vi "用户管理.vi"(6 "用户名的顺序":u16, 8 "用户类别":u8, 9 "管理人员1+密码":string[][](array[string]), 10 "操作人员0+密码":string[][](array[string]), 11 "密码文件路径":path=path "E:/LabVIEW Data/盾构/default") -> (0 "用户类别-out":u8, 1 "管理人员1+密码-out":string[][](array[string]), 2 "操作人员0+密码-out":string[][](array[string]), 3 "用户信息":string, 5 "用户名的顺序-out":u16)   [LabVIEW 2018]
panel:
  out "数值-当前用户名":u16
  out "数值-当前用户类别":u8
  in  "切换用户":bool
  in  "返回":bool
  in  "修改密码":bool
  in  "删除":bool
  in  "增加":bool
  in  "请输入密码":string
  in  "用户名":u16(ring) items=["1", "2"]
  in  "用户类别":u8(ring) items=["操作人员", "管理人员"]
  out "当前用户类别":string
  out "当前用户名":string
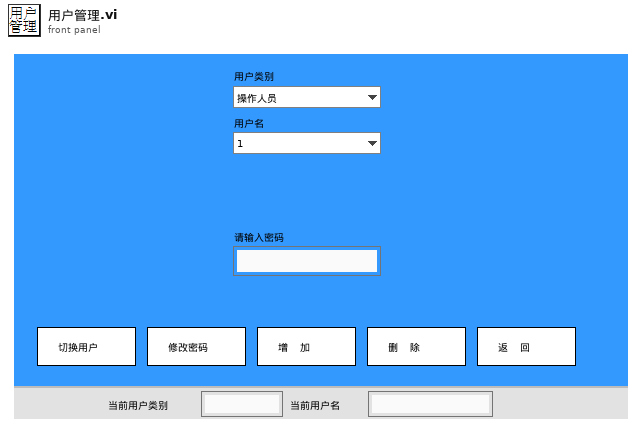
[diagram p1: front panel]
types:
  T1 = cluster{"数值-当前用户类别":u8, "当前用户类别":string, "数值-当前用户名":u16, "当前用户名":string}
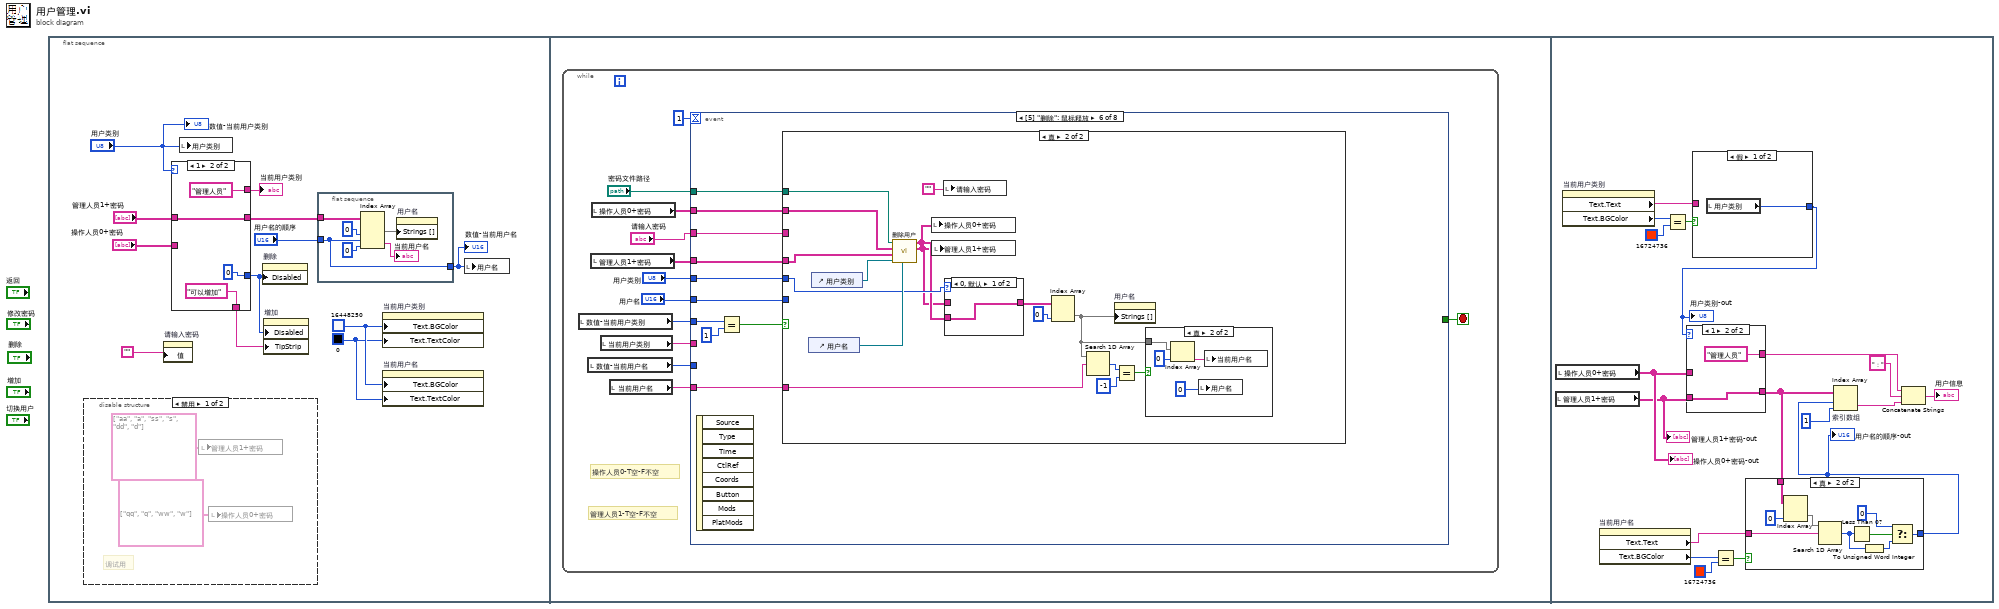
[diagram p0: block diagram]
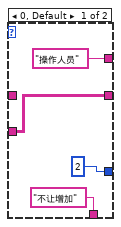
[diagram p3: hidden frame]
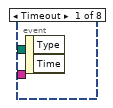
[diagram p4: hidden frame]
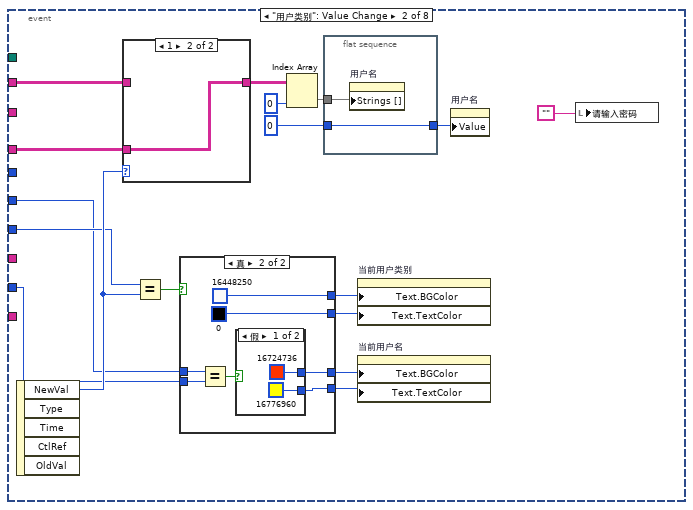
[diagram p5: hidden frame]
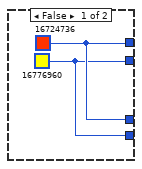
[diagram p6: hidden frame]
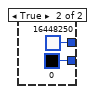
[diagram p7: hidden frame]
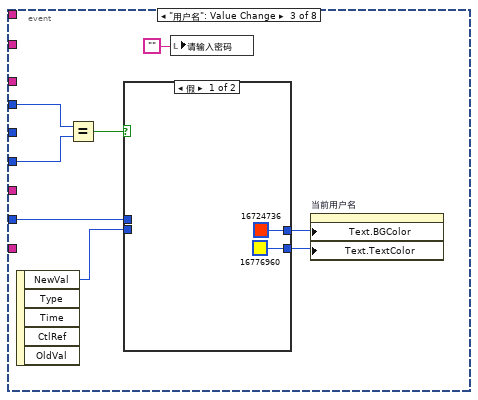
[diagram p9: hidden frame]
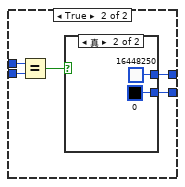
[diagram p10: hidden frame]
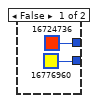
[diagram p11: hidden frame]
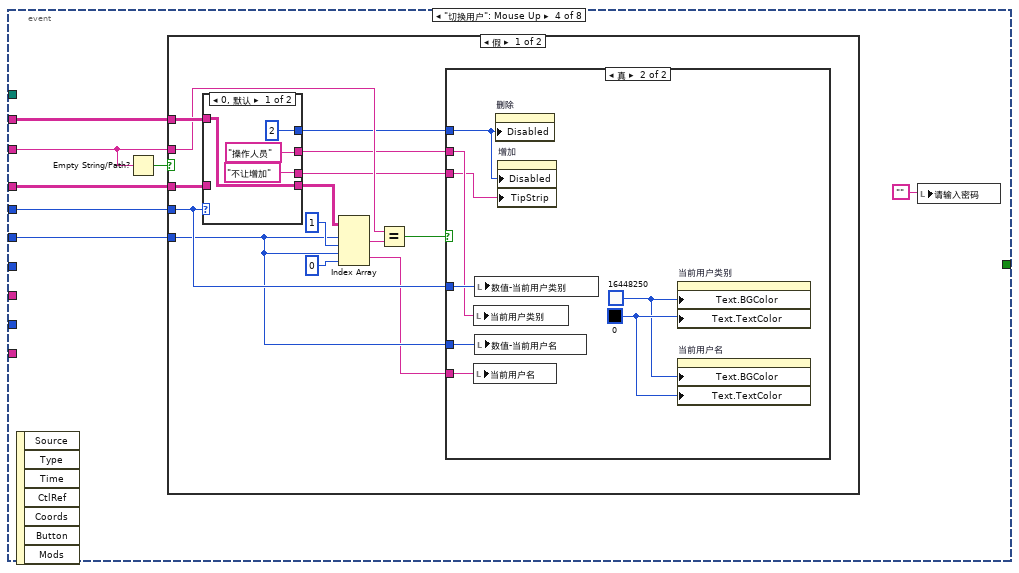
[diagram p12: hidden frame]
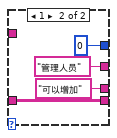
[diagram p14: hidden frame]
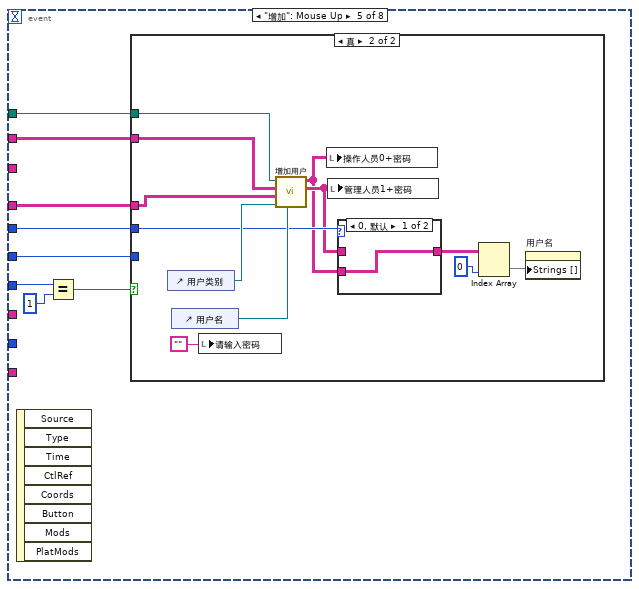
[diagram p16: hidden frame]
diagram:
  n1 = flat-sequence {
    frame #0 {
      w3 = u32 16448250 ("前")
      w2 = u32 0 ("颜色盒")
      n2 = disable-structure shown="禁用" {
        frame Disabled {
          # "调试用"
          n3 = local write "管理人员1+密码"(string[][] [["aa", "a"], ["ss", "s"], ["dd", "d"]] ("管理人员1+密码")) -> ()
          n4 = local write "操作人员0+密码"(string[][] [["qq", "q"], ["ww", "w"]] ("管理人员1+密码")) -> ()
        }
        frame Enabled {
        }
      }
      n5 = property on="请输入密码" class="Str"("值"="") -> ()  [unwired: 2 in, 2 out]
      n6 = case shown="1" "用户类别" {
        tunnel: ["操作人员" "管理人员"] -> w11
        tunnel: "管理人员1+密码" -> [_ w27]
        tunnel: [w23 w27] -> w10
        tunnel: "操作人员0+密码" -> [w23 _]
        tunnel: [u8 2 ("禁用") u8 0 ("禁用")] -> w6
        tunnel: ["不让增加" "可以增加"] -> w1
        frame 0, Default {
        }
        frame 1 {
        }
      }
      "当前用户类别" <- w11
      n7 = local write "用户类别"("用户类别") -> ()
      n8 = property on="删除" class="Bool (严格)"("Disabled"=w6) -> ()  [unwired: 2 in, 2 out]
      n9 = property on="增加" class="Bool (严格)"("Disabled"=w6, "TipStrip"=w1) -> ()  [unwired: 2 in, 2 out]
      n10 = flat-sequence {
        tunnel: w10 -> [w19]
        tunnel: "用户名的顺序" -> [w15]
        tunnel: [w15] -> w8
        frame #0 {
          n11 = Index Array(array=w19, index (col) #1=0 ("禁用的索引 (col)"), index (row) #2=w15, index (col) #2=0 ("禁用的索引 (col)")) -> (element #1=w17:string[], element #2=→"当前用户名":string)  [unwired: 1 in]
          n12 = property on="用户名" class="Ring (严格)"("Strings []"=w17) -> ()  [unwired: 2 in, 2 out]
        }
      }
      n13 = property on="当前用户类别" class="字符串"("Text.BGColor"=w3, "Text.TextColor"=w2) -> ()  [unwired: 2 in, 2 out]
      n14 = property on="当前用户名" class="字符串"("Text.BGColor"=w3, "Text.TextColor"=w2) -> ()  [unwired: 2 in, 2 out]
      n15 = local write "用户名"(w8) -> ()
      "数值-当前用户类别" <- "用户类别"
      "数值-当前用户名" <- w8
    }
    frame #1 {
      n16 = while {
        stop <- w40 stop-if-true
        # "管理人员1-T空-F不空"
        # "操作人员0-T空-F不空"
        n17 = local read "数值-当前用户类别"() -> (w33:u8)
        n18 = local read "数值-当前用户名"() -> (w31:u16)
        n19 = local read "管理人员1+密码"() -> (w36:string[][])
        n20 = local read "操作人员0+密码"() -> (w37:string[][])
        n21 = local read "当前用户类别"() -> (w32:string)
        n22 = local read "当前用户名"() -> (w30:string)
        n23 = event shown="[5] \"删除\": 鼠标释放" {
          selector: _ -> [_ _ _ _ _ _ _ _]
          dyn-events: _ -> [_ _ _ _ _ _ _ _]
          timeout: 1 -> [_ _ _ _ _ _ _ _]
          tunnel: [_ _ _ _ _ _ _ TRUE] -> w40
          tunnel: w37 -> [_ w57 _ w98 w138 w162 w194 _]
          tunnel: w36 -> [_ w54 _ w97 w137 w161 w193 _]
          tunnel: "用户类别" -> [_ _ w78 w100 w136 w160 _ _]
          tunnel: "用户名" -> [_ w43 _ w99 w135 w159 _ _]
          tunnel: "密码文件路径" -> [_ _ _ _ w131 w154 w195 _]
          tunnel: "请输入密码" -> [_ _ _ w96 _ w158 _ _]
          tunnel: w33 -> [_ w49 w77 _ w134 w157 w189 _]
          tunnel: w32 -> [_ _ _ _ _ _ w188 _]
          tunnel: w31 -> [_ w42 w79 _ _ _ w187 _]
          tunnel: w30 -> [_ _ _ _ _ w153 w186 _]
          event Timeout {
            n24 = event-data() -> ()  [unwired: 1 in, 2 out]
          }
          event "用户类别": Value Change {
            n25 = event-data() -> ("NewVal"=w50:u8)  [unwired: 1 in, 4 out]
            n26 = case shown="1" w50 {
              tunnel: w57 -> [w73 _]
              tunnel: [w73 w74] -> w55
              tunnel: w54 -> [_ w74]
              frame 0, Default {
              }
              frame 1 {
              }
            }
            n27 = Equal?(x=w49, y=w50) -> (x = y?=w48:bool)
            n28 = case shown="真" w48 {
              tunnel: [w59 u32 16448250 ("前")] -> w47
              tunnel: [w58 u32 0 ("颜色盒")] -> w46
              tunnel: [w59 w61] -> w45
              tunnel: [w58 w60] -> w44
              tunnel: w43 -> [_ w63]
              tunnel: w42 -> [_ w62]
              frame False {
                w59 = u32 16724736 ("前")
                w58 = u32 16776960 ("颜色盒")
              }
              frame True {
                n29 = Equal?(x=w63, y=w62) -> (x = y?=w64:bool)
                n30 = case shown="假" w64 {
                  tunnel: [u32 16724736 ("前") u32 16448250 ("前")] -> w61
                  tunnel: [u32 16776960 ("颜色盒") u32 0 ("颜色盒")] -> w60
                  frame False {
                  }
                  frame True {
                  }
                }
              }
            }
            n31 = Index Array(array=w55, index (col)=0 ("禁用的索引 (col)")) -> (element=w56:string[])  [unwired: 1 in]
            n32 = flat-sequence {
              tunnel: w56 -> [w72]
              tunnel: [w71] -> w51
              tunnel: u16 0 ("禁用的索引 (col)") -> [w71]
              frame #0 {
                n33 = property on="用户名" class="Ring (严格)"("Strings []"=w72) -> ()  [unwired: 2 in, 2 out]
              }
            }
            n34 = property on="当前用户类别" class="字符串"("Text.BGColor"=w47, "Text.TextColor"=w46) -> ()  [unwired: 2 in, 2 out]
            n35 = property on="当前用户名" class="字符串"("Text.BGColor"=w45, "Text.TextColor"=w44) -> ()  [unwired: 2 in, 2 out]
            n36 = property on="用户名" class="Ring (严格)"("Value"=w51) -> ()  [unwired: 2 in, 2 out]
            n37 = local write "请输入密码"("") -> ()
          }
          event "用户名": Value Change {
            n38 = event-data() -> ("NewVal"=w82:u16)  [unwired: 1 in, 4 out]
            n39 = Equal?(x=w78, y=w77) -> (x = y?=w76:bool)
            n40 = case shown="假" w76 {
              tunnel: w82 -> [_ w89]
              tunnel: [u32 16724736 ("前") w87] -> w81
              tunnel: [u32 16776960 ("颜色盒") w86] -> w80
              tunnel: w79 -> [_ w85]
              frame False {
              }
              frame True {
                n41 = Equal?(x=w85, y=w89) -> (x = y?=w88:bool)
                n42 = case shown="真" w88 {
                  tunnel: [u32 16724736 ("前") u32 16448250 ("前")] -> w87
                  tunnel: [u32 16776960 ("颜色盒") u32 0 ("颜色盒")] -> w86
                  frame False {
                  }
                  frame True {
                  }
                }
              }
            }
            n43 = local write "请输入密码"("") -> ()
            n44 = property on="当前用户名" class="字符串"("Text.BGColor"=w81, "Text.TextColor"=w80) -> ()  [unwired: 2 in, 2 out]
          }
          event "切换用户": Mouse Up {
            n45 = event-data() -> ()  [unwired: 1 in, 7 out]
            n46 = Empty String/Path?(string/path=w96) -> (empty?=w94:bool)
            n47 = case shown="假" w94 {
              tunnel: w100 -> [w107 _]
              tunnel: w99 -> [w105 _]
              tunnel: w98 -> [w114 _]
              tunnel: w97 -> [w113 _]
              tunnel: w96 -> [w109 _]
              frame False {
                n48 = case shown="0, 默认" w107 {
                  tunnel: w114 -> [w126 _]
                  tunnel: w113 -> [_ w130]
                  tunnel: [w126 w130] -> w110
                  tunnel: ["操作人员" "管理人员"] -> w103
                  tunnel: [u8 2 ("禁用") u8 0 ("禁用")] -> w102
                  tunnel: ["不让增加" "可以增加"] -> w101
                  frame 0, Default {
                  }
                  frame 1 {
                  }
                }
                n49 = Index Array(array=w110, index (row) #1=w105, index (col) #1=1 ("禁用的索引 (col)"), index (row) #2=w105, index (col) #2=0 ("禁用的索引 (col)")) -> (element #1=w111:string, element #2=w104:string)
                n50 = Equal?(x=w109, y=w111) -> (x = y?=w108:bool)
                n51 = case shown="真" w108 {
                  tunnel: w107 -> [_ w122]
                  tunnel: w105 -> [_ w121]
                  tunnel: w104 -> [_ w120]
                  tunnel: w103 -> [_ w119]
                  tunnel: w102 -> [_ w116]
                  tunnel: w101 -> [_ w115]
                  frame False {
                  }
                  frame True {
                    w117 = u32 16448250 ("前")
                    w118 = u32 0 ("颜色盒")
                    n52 = local write "当前用户类别"(w119) -> ()
                    n53 = local write "当前用户名"(w120) -> ()
                    n54 = local write "数值-当前用户类别"(w122) -> ()
                    n55 = local write "数值-当前用户名"(w121) -> ()
                    n56 = property on="删除" class="Bool (严格)"("Disabled"=w116) -> ()  [unwired: 2 in, 2 out]
                    n57 = property on="增加" class="Bool (严格)"("Disabled"=w116, "TipStrip"=w115) -> ()  [unwired: 2 in, 2 out]
                    n58 = property on="当前用户类别" class="字符串"("Text.BGColor"=w117, "Text.TextColor"=w118) -> ()  [unwired: 2 in, 2 out]
                    n59 = property on="当前用户名" class="字符串"("Text.BGColor"=w117, "Text.TextColor"=w118) -> ()  [unwired: 2 in, 2 out]
                  }
                }
              }
              frame True {
              }
            }
            n60 = local write "请输入密码"("") -> ()
          }
          event "增加": Mouse Up {
            n61 = event-data() -> ()  [unwired: 1 in, 8 out]
            n62 = Equal?(x=w134, y=u8 1) -> (x = y?=w132:bool)
            n63 = case shown="真" w132 {
              tunnel: w138 -> [_ w149]
              tunnel: w137 -> [_ w148]
              tunnel: w136 -> [_ w144]
              tunnel: w135 -> [_ _]
              tunnel: w131 -> [_ w150]
              frame False {
              }
              frame True {
                n64 = control-ref of="用户类别"() -> (w147:refnum<vi>)
                n65 = control-ref of="用户名"() -> (w146:refnum<vi>)
                n66 = local write "请输入密码"("") -> ()
                n67 = call "增加用户.vi"("用户名-refnum-in"=w146, "用户类别-refnum-in"=w147, "管理人员1+密码"=w148, "操作人员0+密码"=w149, "密码文件路径"=w150) -> ("管理人员1+密码_out"=w143:string[][], "操作人员0+密码_out"=w142:string[][])  [unwired: 5 in]
                n68 = local write "操作人员0+密码"(w142) -> ()
                n69 = local write "管理人员1+密码"(w143) -> ()
                n70 = case shown="0, 默认" w144 {
                  tunnel: w143 -> [_ w152]
                  tunnel: [w151 w152] -> w139
                  tunnel: w142 -> [w151 _]
                  frame 0, Default {
                  }
                  frame 1 {
                  }
                }
                n71 = Index Array(array=w139, index (col)=0 ("禁用的索引 (col)")) -> (element=w140:string[])  [unwired: 1 in]
                n72 = property on="用户名" class="Ring (严格)"("Strings []"=w140) -> ()  [unwired: 2 in, 2 out]
              }
            }
          }
          event "删除": Mouse Up {
            n73 = event-data() -> ()  [unwired: 1 in, 8 out]
            n74 = Equal?(x=w157, y=u8 1) -> (x = y?=w155:bool)
            n75 = case shown="真" w155 {
              tunnel: w162 -> [_ w177]
              tunnel: w161 -> [_ w176]
              tunnel: w160 -> [_ w170]
              tunnel: w159 -> [_ _]
              tunnel: w158 -> [_ _]
              tunnel: w154 -> [_ w178]
              tunnel: w153 -> [_ w167]
              frame False {
              }
              frame True {
                n76 = control-ref of="用户名"() -> (w174:refnum<vi>)
                n77 = control-ref of="用户类别"() -> (w175:refnum<vi>)
                n78 = call "删除用户.vi"("用户名-refnum-in"=w174, "用户类别-refnum-in"=w175, "管理人员1+密码"=w176, "操作人员0+密码"=w177, "密码文件路径"=w178) -> ("管理人员1+密码_out"=w168:string[][], "操作人员0+密码_out"=w169:string[][])  [unwired: 5 in]
                n79 = local write "操作人员0+密码"(w169) -> ()
                n80 = local write "管理人员1+密码"(w168) -> ()
                n81 = local write "请输入密码"("") -> ()
                n82 = case shown="0, 默认" w170 {
                  tunnel: w168 -> [_ w184]
                  tunnel: [w183 w184] -> w171
                  tunnel: w169 -> [w183 _]
                  frame 0, Default {
                  }
                  frame 1 {
                  }
                }
                n83 = Index Array(array=w171, index (col)=0 ("禁用的索引 (col)")) -> (element=w163:string[])  [unwired: 1 in]
                n84 = Search 1D Array(1D array=w163, element=w167) -> (index of element=w166:i32)  [unwired: 1 in]
                n85 = property on="用户名" class="Ring (严格)"("Strings []"=w163) -> ()  [unwired: 2 in, 2 out]
                n86 = Equal?(x=w166, y=-1) -> (x = y?=w164:bool)
                n87 = case shown="真" w164 {
                  tunnel: w163 -> [_ w182]
                  frame False {
                  }
                  frame True {
                    n88 = Index Array(array=w182, index=0 ("索引")) -> (element=w181:string)
                    n89 = local write "用户名"(u16 0 ("索引")) -> ()
                    n90 = local write "当前用户名"(w181) -> ()
                  }
                }
              }
            }
          }
          event "修改密码": Mouse Up {
            n91 = event-data() -> ()  [unwired: 1 in, 7 out]
            n92 = Bundle("数值-当前用户类别"=w189, "当前用户类别"=w188, "数值-当前用户名"=w187, "当前用户名"=w186) -> (w190:T1)  [unwired: 1 in]
            n93 = call "修改密码.vi"("当前用户信息"=w190, "管理人员1+密码"=w193, "操作人员0+密码"=w194, "密码文件路径"=w195) -> ("管理人员1+密码_out"=w191:string[][], "操作人员0+密码_out"=w192:string[][])  [unwired: 6 in]
            n94 = local write "管理人员1+密码"(w191) -> ()
            n95 = local write "操作人员0+密码"(w192) -> ()
            n96 = local write "请输入密码"("") -> ()
          }
          event "返回": Mouse Up; Panel Close {
            n97 = event-data() -> ()  [unwired: 1 in, 3 out]
            n98 = local write "请输入密码"("") -> ()
          }
        }
      }
    }
    frame #2 {
      n99 = local read "管理人员1+密码"() -> (w210:string[][])
      "管理人员1+密码-out" <- w210
      n100 = local read "操作人员0+密码"() -> (w211:string[][])
      "操作人员0+密码-out" <- w211
      n101 = property on="当前用户类别" class="字符串"() -> ("Text.Text"=w205:string, "Text.BGColor"=w208:u32)  [unwired: 2 in, 2 out]
      n102 = property on="当前用户名" class="字符串"() -> ("Text.Text"=w199:string, "Text.BGColor"=w202:u32)  [unwired: 2 in, 2 out]
      n103 = Equal?(x=w208, y=u32 16724736 ("前")) -> (x = y?=w206:bool)
      n104 = case shown="假" w206 {
        tunnel: w205 -> [_ w232]
        tunnel: [w226 w227] -> w204
        frame False {
          n105 = local read "用户类别"() -> (w226:u8)
        }
        frame True {
          w230 = u8 1 items=["操作人员", "管理人员"] ("用户类别")
          w228 = u8 0 items=["操作人员", "管理人员"] ("用户类别")
          n106 = Equal?(x=w232, y="管理人员") -> (x = y?=w229:bool)
          n107 = Select(t=w230, s=w229, f=w228) -> (s? t:f=w227:u8)
        }
      }
      "用户类别-out" <- w204
      n108 = case shown="1" w204 {
        tunnel: ["操作人员" "管理人员"] -> w212
        tunnel: w210 -> [_ w235]
        tunnel: [w233 w235] -> w201
        tunnel: w211 -> [w233 _]
        frame 0, Default {
        }
        frame 1 {
        }
      }
      n109 = Equal?(x=w202, y=u32 16724736 ("前")) -> (x = y?=w200:bool)
      n110 = case shown="真" w200 {
        tunnel: w201 -> [_ w224]
        tunnel: w199 -> [_ w222]
        tunnel: [w216 w217] -> w198
        frame False {
          n111 = local read "用户名"() -> (w216:u16)
        }
        frame True {
          n112 = Index Array(array=w224, index (col)=0 ("禁用的索引 (col)")) -> (element=w223:string[])  [unwired: 1 in]
          n113 = Search 1D Array(1D array=w223, element=w222) -> (index of element=w219:i32)  [unwired: 1 in]
          n114 = Less Than 0?(x=w219) -> (x < 0?=w221:bool)
          n115 = To Unsigned Word Integer(number=w219) -> (unsigned 16bit integer=w218:u16)
          n116 = Select(t=u16 0 ("用户名的顺序-out"), s=w221, f=w218) -> (s? t:f=w217:u16)
        }
      }
      "用户名的顺序-out" <- w198
      n117 = Index Array "索引数组"(array=w201, index (row)=w198, index (col)=1 ("禁用的索引 (col)")) -> (element=w215:string)
      n118 = Concatenate Strings(w212, "：", w215) -> (→"用户信息":string)
    }
  }
